vi "Roaming.vi"() -> ()   [LabVIEW 2013]
uses:
  <vilib>/Platform/TimedLoop/XDataNode/timing_clust.ctl
  <vilib>/Platform/TimedLoop/XDataNode/nitl_modes.ctl
  <vilib>/Platform/TimedLoop/XDataNode/wakeup.ctl
  <vilib>/Instr/_visa.llb/VISA Configure Serial Port (Instr).vi
  <vilib>/FPGAPlugInAG/sbRIO-9642/niLvFpga_Open_sbRIO-9642.vi
  <vilib>/rvi/interface/common/dynamic/niFpgaDynamicAddResources.vi
  <vilib>/rvi/interface/common/niFpgaWaitOnOcc.vi
  <vilib>/Utility/error.llb/Error Cluster From Error Code.vi
  <vilib>/rvi/errors/niLvFpgaAdjustHostInterfaceError.vi
  <vilib>/Platform/TimedLoop/XDataNode/XDataNode.xnode
  <vilib>/rvi/interface/nirviOpenFPGA/nirviOpenFPGA.xnode
  FPGA Bitfiles/NatesProject1_FPGATarget_FPGAConfig_gDHlPw7zMRU.lvbitx
  FPGA Config.vi
  <vilib>/rvi/interface/nirviReadWriteControl/nirviReadWriteControl.xnode
  <vilib>/robotics/Utilities/Scan Angles/NI_Robotics_Scan Angles.lvlib
  <vilib>/Platform/TimedLoop/XDataNode/XDNodeRunTimeDep.lvlib
  NiFpgaLv.dll
  <vilib>/rvi/interface/Simulation/niFpgaSimulationCallBeginRW.vi
panel:
  out "angle change (scaled)":dbl
  out "velocity change (scaled)":dbl
  out "angle change":dbl
  out "velocity change":dbl
  out "write buffer 2":string
  out "error out":errorcluster
  out "write buffer":string
  in  "VISA resource name":refnum<visa-resource-name>
  out "Sensor Data":cluster{"angles (deg)":dbl[], "distances":dbl[]}(graph)
  out "Front Sensor\nDistance\n(m)":dbl(slide) scale=0.0..2.0
  in  "stop":bool
  out "ModA/AI0":fxp<+/-,26,5>
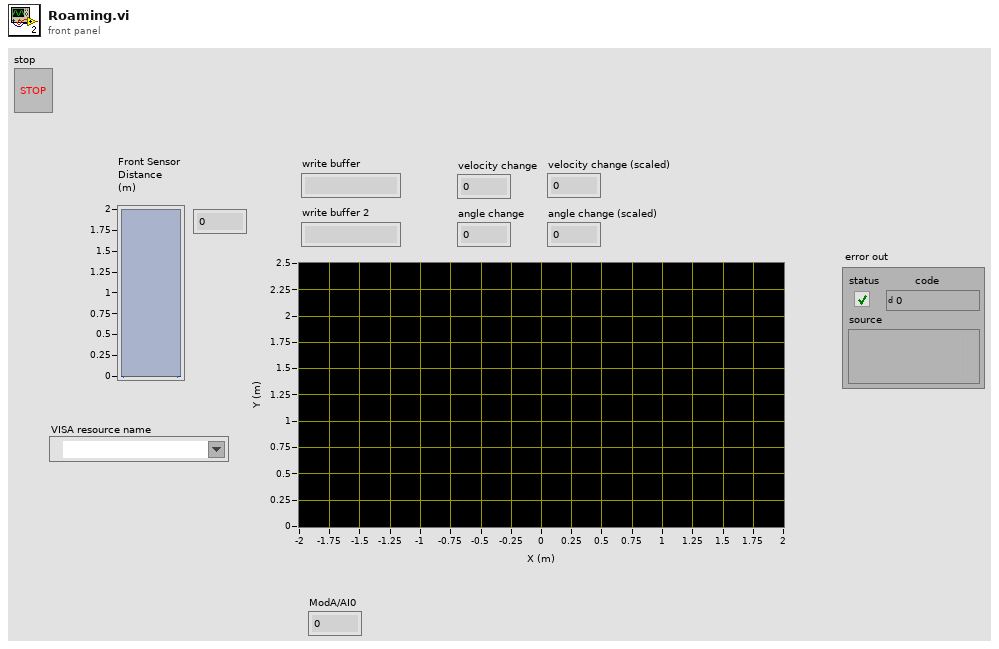
[diagram p1: front panel]
types:
  T1 = typedef "XDNodeRunTimeDep.lvlib/timing_clust.ctl" = cluster{"Expected End [f-1]":u64, "Actual End [f-1]":u64, "Finished Late? [f-1]":bool, "Expected End [i-1]":u64, "Actual End [i-1]":u64, "Finished Late? [i-1]":bool, "Expected Start [i]":u64, "Actual Start [i]":u64, "Expected Start [f]":u64, "Actual Start [f]":u64, "Source Name":string, "Structure Name":string, "Period":i64, "Deadline":i64, "Offset":i64, "Start":i64, "Priority":i32, "Timeout":i32, "Mode":T2, "Wakeup Reason":T3, "Error":errorcluster, "Source Type":string, "Secondary Source Type":string, "Global End Time":u64, "Global Start Time":u64, "Frame Duration":u64, "Iteration Duration":u64, "Assigned CPU":i32, "I/O Scan Engine Mode":u32}
  T2 = typedef "XDNodeRunTimeDep.lvlib/nitl_modes.ctl" = enum32{"No Change", "Process missed periods, maintain original phase", "Discard missed periods, maintain original phase", "Process missed periods, ignore original phase", "Discard missed periods, ignore original phase"}
  T3 = typedef "XDNodeRunTimeDep.lvlib/wakeup.ctl" = enum32{"Normal", "Aborted", "Asynchronous wakeup", "Timing source error", "Timed loop error", "Timeout"}
  T4 = typedef "NI_Robotics_Scan Angles.lvlib/Scan Angle Data.ctl" = cluster{"angles":dbl[], "distances":dbl[], "current index":i32, "previous index":i32}
  T5 = cluster{"steering frame velocity[0]":dbl, "steering frame velocity[1]":dbl, "steering frame velocity[2]":dbl, "steering frame velocity[3]":dbl, "steering frame velocity[4]":dbl, "steering frame velocity[5]":dbl, "steering frame velocity[6]":dbl, "steering frame velocity[7]":dbl, "steering frame velocity[8]":dbl}
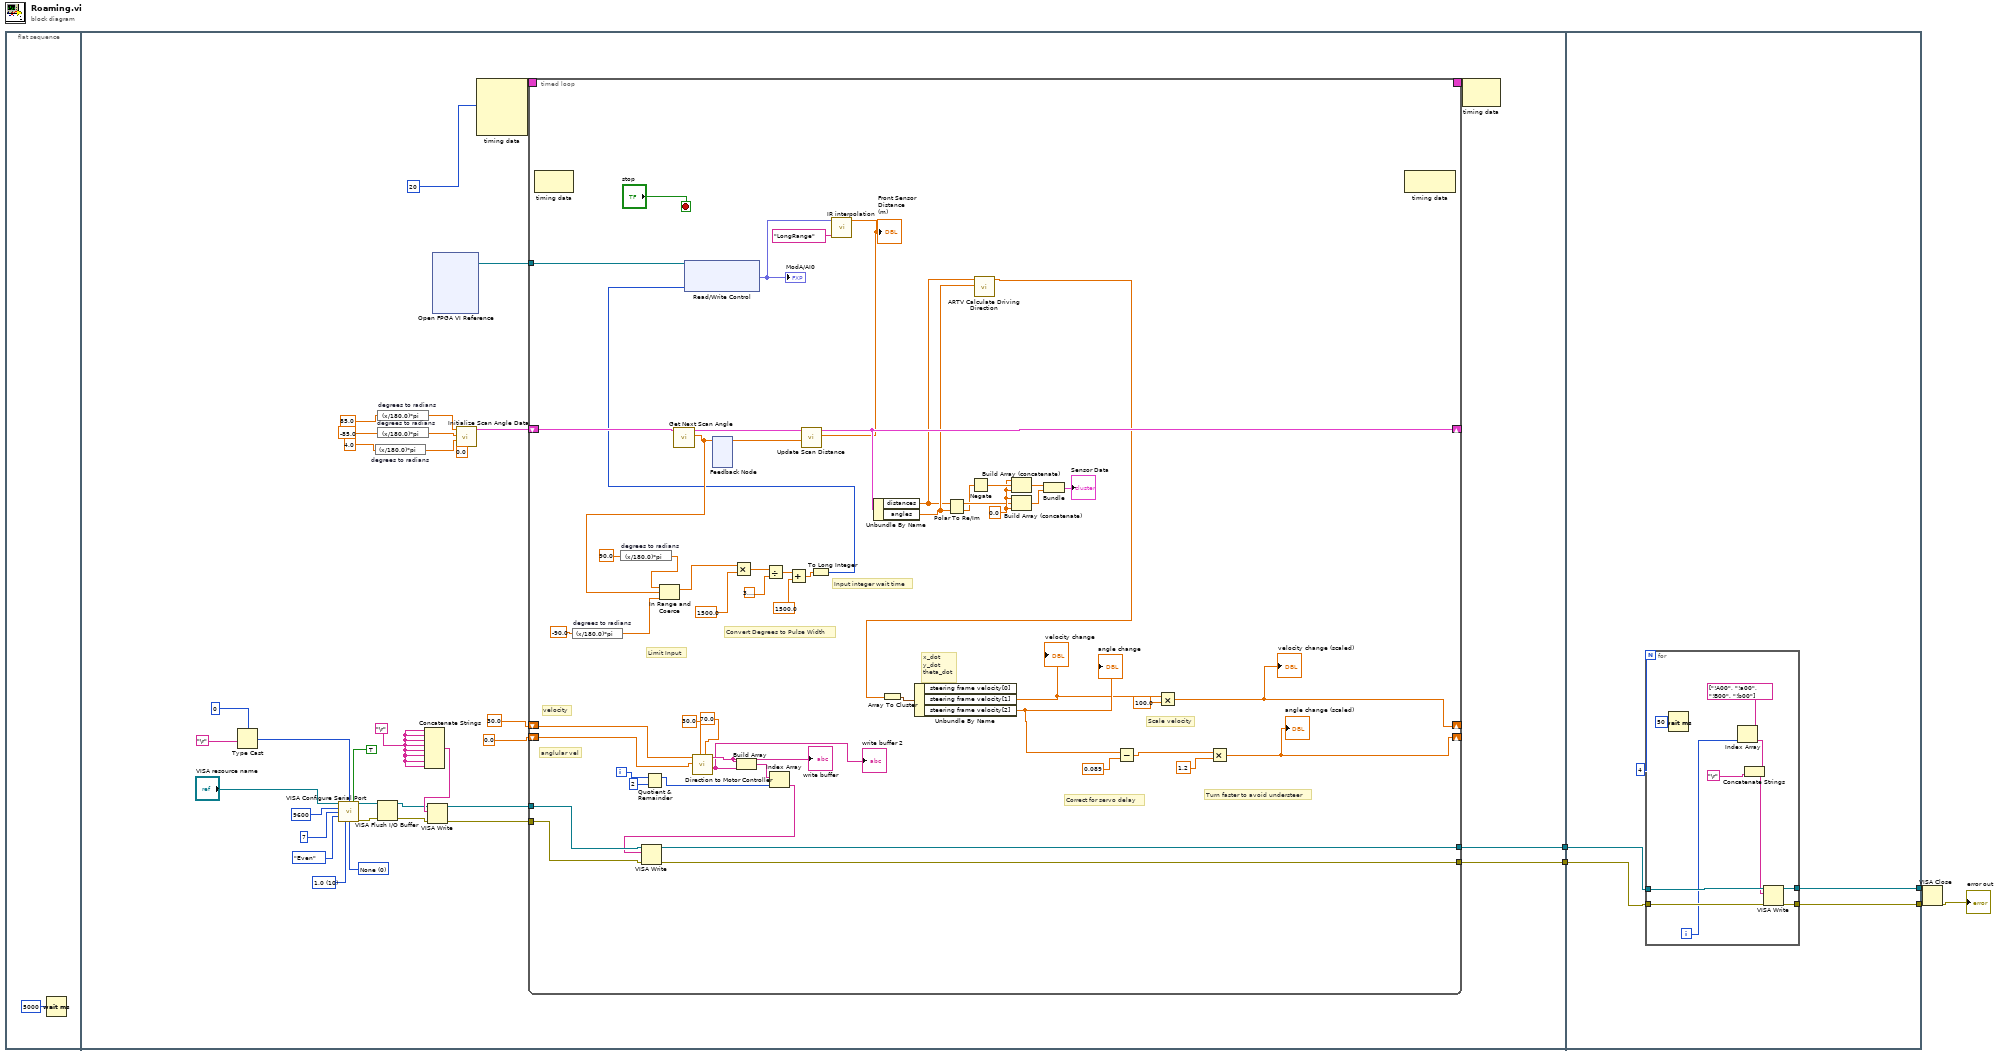
[diagram p0: block diagram]
diagram:
  n1 = flat-sequence {
    tunnel: [w10] -> w4
    tunnel: [w9] -> w3
    tunnel: w4 -> [w106]
    tunnel: w3 -> [w105]
    tunnel: [w104] -> w2
    tunnel: [w103] -> w1
    frame #0 {
      n2 = Wait (ms)(milliseconds to wait=u32 5000) -> ()  [unwired: 1 out]
    }
    frame #1 {
      w16 = "\r"
      w23 = u16 0 items=["None", "XON/XOFF", "RTS/CTS", "XON/XOFF & RTS/CTS", "DTR/DSR", "XON/XOFF & DTR/DSR"] ("flow control (0:none)")
      w24 = u16 10 items=["1.0"=10, "1.5"=15, "2.0"=20] ("stop bits (10: 1 bit)")
      n3 = Type Cast(type=0, x="\r") -> (*(type *) &x=w19:i32)
      n4 = call-poly "VISA Configure Serial Port"("VISA resource name"="VISA resource name", "termination char\n(0xA = '\\n' = LF)"=w19, "Enable Termination\nChar (T)"=TRUE ("Enable Termination\nChar (T)"), "baud rate (9600)"=u32 9600, "data bits (8)"=u16 7, "parity (0:none)"=enum16{"None", "Odd", "Even", "Mark", "Space"}."Even", "stop bits (10: 1 bit)"=w24, "flow control (0:none)"=w23) -> ("VISA resource name out"=w17:refnum<visa-resource-name>, "error out"=w18:errorcluster)  [unwired: 6 in]
      n5 = expression code="(x/180.0)*pi" "degrees to radians"(4.0 ("scan angle")) -> (w31:dbl)
      n6 = VISA Flush I/O Buffer(VISA resource name=w17, error in (no error)=w18) -> (VISA resource name out=w14:refnum<visa-resource-name>, error out=w13:errorcluster)  [unwired: 1 in]
      n7 = expression code="(x/180.0)*pi" "degrees to radians"(85.0 ("max angle")) -> (w33:dbl)
      n8 = expression code="(x/180.0)*pi" "degrees to radians"(-85.0 ("min angle")) -> (w32:dbl)
      n9 = Concatenate Strings(w16, w16, w16, w16, w16, w16, w16, w16) -> (w15:string)
      n10 = VISA Write(VISA resource name=w14, write buffer=w15, error in (no error)=w13) -> (VISA resource name out=w12:refnum<visa-resource-name>, error out=w11:errorcluster)  [unwired: 1 out]
      n11 = xnode "Open FPGA VI Reference"() -> ("FPGA VI Reference Out"=w38:refnum<k20>)  [unwired: 2 in, 1 out]
      n12 = call <vilib>:"Initialize Scan Angle Data.vi"("initial angle (0)"=0.0, "scan angle"=w31, "min angle"=w32, "max angle"=w33) -> ("scan angles"=w36:T4)  [unwired: 6 in, 1 out]
      n13 = node-c288(i64 20 ("Period")) -> (w40:T1)  [unwired: 3 in]
      n14 = timed-loop {
        tunnel: w38 -> [w93]
        shift-right: [w69] -> _
        shift-left: w36 -> [w90]
        timing: w40 -> [_]
        timing-out: [_] -> w39
        tunnel: w12 -> [w66]
        tunnel: w11 -> [w65]
        tunnel: [w64] -> w10
        tunnel: [w63] -> w9
        shift-right: [w43] -> _
        shift-left: 0.0 -> [w51]
        shift-right: [w42] -> _
        shift-left: 30.0 -> [w56]
        i -> [w59]
        stop <- "stop" stop-if-true
        w74 = 0.0 ("element")
        # "Scale velocity"
        # "Turn faster to avoid understeer"
        # "Correct for servo delay"
        # "velocity"
        # "anglular vel"
        # "x_dot\ny_dot\ntheta_dot"
        # "Input integer wait time"
        # "Convert Degrees to Pulse Width"
        # "Limit Input"
        n15 = node-c288() -> ()  [unwired: 1 in, 1 out]
        n16 = expression code="(x/180.0)*pi" "degrees to radians"(-90.0 ("lower limit")) -> (w78:dbl)
        n17 = expression code="(x/180.0)*pi" "degrees to radians"(90.0 ("upper limit")) -> (w77:dbl)
        n18 = Quotient & Remainder(x=w59, y=2) -> (x-y*floor(x/y)=w57:i32)  [unwired: 1 out]
        n19 = call <vilib>:"Get Next Scan Angle.vi"("scan angles in"=w90) -> ("new angle"=w83:dbl, "scan angles out"=w92:T4)  [unwired: 9 in]
        n20 = In Range and Coerce(upper limit=w77, x=w83, lower limit=w78) -> (coerced(x)=w89:dbl)  [unwired: 1 out]
        n21 = call "Direction to Motor Controller.vi"("Turn Percent Limit"=70.0, "Percent Limit"=30.0, "Angular vel (rad/s)"=w51, "Vel (m/s)"=w56) -> ("Turn Direction"=w53:string, "Forward Direction"=w54:string)  [unwired: 6 in]
        "write buffer" <- w54
        "write buffer 2" <- w53
        n22 = feedback #1() -> (w91:dbl)  [unwired: 1 in]
        n23 = feedback-in #1(w83) -> ()
        n24 = Multiply(x=w89, y=1500.0) -> (x*y=w88:dbl)
        n25 = Build Array(w54, w53) -> (w60:string[])
        n26 = Divide(x=w88, y=3.141592653589793) -> (x/y=w86:dbl)
        n27 = Index Array(array=w60, index=w57) -> (element=w55:string)
        n28 = VISA Write(VISA resource name=w66, write buffer=w55, error in (no error)=w65) -> (VISA resource name out=w64:refnum<visa-resource-name>, error out=w63:errorcluster)  [unwired: 1 out]
        n29 = Add(x=w86, y=1500.0) -> (x+y=w85:dbl)
        n30 = To Long Integer(number=w85) -> (32bit integer=w82:i32)
        n31 = xnode "Read/Write Control"("FPGA VI Reference In"=w93, "Pulse Width(uSec)"=w82) -> ("ModA/AI1"=w95:fxp<+/-,26,5>)  [unwired: 1 in, 2 out]
        "ModA/AI0" <- w95
        n32 = call "IR interpolation.vi"("IR Sensor Type"="LongRange", "x value"=w95) -> ("interpolation value"=w41:dbl)  [unwired: 9 in]
        "Front Sensor\nDistance\n(m)" <- w41
        n33 = call <vilib>:"Update Scan Distance.vi"("scan angle"=w91, "new scan distance"=w41, "scan angles in"=w92) -> ("scan angles out"=w69:T4)  [unwired: 8 in]
        n34 = Unbundle By Name(w69) -> ("distances"=w67:dbl[], "angles"=w68:dbl[])
        n35 = Polar To Re/Im(2:w68, 3:w67) -> (0:w71:dbl[], 1:w72:dbl[])
        n36 = Negate(x=w71) -> (-x=w76:dbl[])
        n37 = call "ARTV Calculate Driving Direction.vi"("obstacle angles (rad)"=w68, "obstacle distances (m)"=w67) -> ("steering frame velocity"=w62:dbl[])  [unwired: 8 in, 1 out]
        n38 = Array To Cluster(array=w62) -> (cluster=w61:T5)
        n39 = Unbundle By Name(w61) -> ("steering frame velocity[1]"=w45:dbl, "steering frame velocity[2]"=w52:dbl)  [unwired: 1 out]
        "velocity change" <- w45
        "angle change" <- w52
        n40 = Build Array (concatenate)(w74, w76, w74) -> (w75:dbl[])
        n41 = Build Array (concatenate)(w74, w72, w74) -> (w73:dbl[])
        n42 = Bundle(w75, w73) -> (→"Sensor Data":cluster{dbl[], dbl[]})  [unwired: 1 in]
        n43 = Subtract(x=w52, y=0.089) -> (x-y=w47:dbl)
        n44 = Multiply(x=w45, y=100.0) -> (x*y=w42:dbl)
        "velocity change (scaled)" <- w42
        n45 = Multiply(x=w47, y=1.2) -> (x*y=w43:dbl)
        "angle change (scaled)" <- w43
        n46 = node-c288() -> ()  [unwired: 1 in, 1 out]
      }
      n47 = node-c288(w39) -> ()  [unwired: 1 out]
    }
    frame #2 {
      n48 = for {
        N: 4 -> [_]
        tunnel: w106 -> [w117]
        tunnel: w105 -> [w116]
        tunnel: [w115] -> w104
        tunnel: [w114] -> w103
        i -> [w112]
        n49 = Wait (ms)(milliseconds to wait=u32 50) -> ()  [unwired: 1 out]
        n50 = Index Array(array=string[] ["!A00", "!a00", "!B00", "!b00"], index=w112) -> (element=w110:string)
        n51 = Concatenate Strings(w110, "\r") -> (w108:string)
        n52 = VISA Write(VISA resource name=w117, write buffer=w108, error in (no error)=w116) -> (VISA resource name out=w115:refnum<visa-resource-name>, error out=w114:errorcluster)  [unwired: 1 out]
      }
    }
  }
  n53 = VISA Close(VISA resource name=w2, error in (no error)=w1) -> (error out=→"error out":errorcluster)
